vi "Make Arrays right length.vi"(1 "Errors":dbl[](array[numeric]), 2 "Data":dbl[](array[numeric])) -> (0 "Errors[1..len(Data)]":dbl[](array[numeric]))   [LabVIEW 2012, in "XY Plot with Error Bars.xctl"]
uses:
  XY Plot with Error Bars.xctl
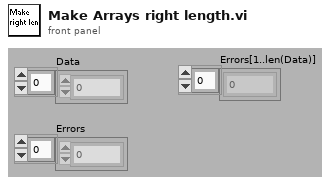
[diagram p1: front panel]
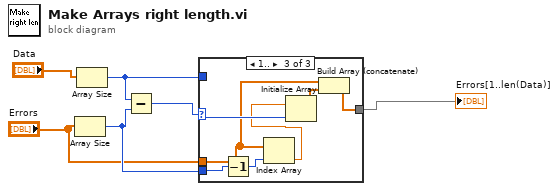
[diagram p0: block diagram]
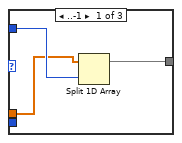
[diagram p2: hidden frame]
diagram:
  n1 = Array Size(array="Errors") -> (size(s)=w4:i32)
  n2 = Array Size(array="Data") -> (size(s)=w2:i32)
  n3 = Subtract(x=w2, y=w4) -> (x-y=w1:i32)
  n4 = case shown="1.." w1 {
    selector: w1 -> [_ _ w15]
    tunnel: w2 -> [w9 _ _]
    tunnel: "Errors" -> [w8 w10 w13]
    tunnel: [w7 w10 w11] -> w5
    tunnel: w4 -> [_ _ w16]
    frame ..-1 {
      n5 = Split 1D Array(array=w8, index=w9) -> (first subarray=w7:dbl[])  [unwired: 1 out]
    }
    frame 0 {
    }
    frame 1.. {
      n6 = Decrement(x=w16) -> (x-1=w17:i32)
      n7 = Index Array(array=w13, index=w17) -> (element=w14:dbl)
      n8 = Initialize Array(w14, w15) -> (w12:dbl[])
      n9 = Build Array (concatenate)(w13, w12) -> (w11:dbl[])
    }
  }
  "Errors[1..len(Data)]" <- w5
